vi "QAM_equalization.vi"() -> ()   [LabVIEW 2010]
doc: "This example demonstrates the implementation of Equalization in an QAM Modulation Demodulation System"
uses:
  <vilib>/AddOns/Modulation/Digital/General/MT Generate QAM System Parameters(M).vi
  <vilib>/measure/masml.llb/ma_sml_Interpolation by Zero Insert (complex input).vi
  <vilib>/addons/Modulation/Digital/General/MT Generate Bits (Galois, PN Order).vi
  <vilib>/AddOns/Modulation/Digital/General/MT Apply Matched Filter (Generic).vi
  <vilib>/AddOns/Modulation/Digital/General/MT Align to Ideal Symbols (Generic).vi
  <vilib>/AddOns/Modulation/Digital/Equalization/MT QAM Feedforward Equalizer (LMS) (Specify coefficients).vi
  <vilib>/AddOns/Modulation/Digital/Demodulation/MT Calculate BER After Trigger (PN Sequence).vi
  <vilib>/addons/Modulation/niDMT.lvlib
  <vilib>/Analysis/NI_AALBase.lvlib
  <vilib>/measure/NI_MAPro.lvlib
  <vilib>/AddOns/Modulation/Digital/General/MT Generate Symbol Map (Rectangular).vi
  <vilib>/AddOns/Modulation/Digital/General/MT Map Bits to QAM Symbols.vi
panel:
  out "pulse shaping filter coefficients":dbl[](graph)
  out "大小 5":i32
  out "大小 4":i32
  out "大小 3":i32
  out "大小 2":i32
  out "大小":i32
  out "Error Out":errorcluster
  in  "Error In":errorcluster
  in  "Reset?":bool
  out "Recovered":i8[](array[numeric])
  out "Message":i8[](array[numeric])
  in  "Equalizer length \n(symbols)":i32=48
  in  "PN Sequence Order":i32=26
  in  "Channel Filter Length\n(symbols)":i32=8
  out "BER Trigger Found Index (Bits)":u32
  out "Optimal Offset (Samples)":dbl format="%.4f"
  in  "Seed In":i32=-1
  out "Modulation Error Ratio (dB)":dbl format="%.2f"
  in  "Training Length\n(symbols)":i32=500
  in  "Channel Filter":T1(ring)=enum."Low-pass"
  out "BER":dbl format="%.4f"
  in  "Eb/N0 (10 dB)":dbl=50.0 format="%.2f"
  in  "Tab Control":T2(tab)=enum."RX Constellation (post equ)"
  in  "autoscale Tx":bool
  out "Constellation Graph (pre equ)":T3(graph)
  in  "Reset action":string="The example VI performs the following actions depending on the\nvalue of the boolean controls Reset? and Retrain Equalizer? :\n\n1. Reset?=TRUE: Reset all internal VIs,initialize equalizer coefficient array to equal the time-delayed dirac delta response {0 0 0... 1 ...0 0 0}, and feed training bits for equalization.\n\n2. Reset?=FALSE, Retrain Equalizer?=TRUE: Reset all receiver side VIs only,continue training the equalizer, and use final equalizer coefficient array from output of previous iteration as initial conditions for equalizer in current iteration\n\n3. Reset?=FALSE, Retrain Equalizer?=FALSE: Continue modulation, demodulation and equalization from previous iteration, while performing equalization in decision directed mode. This simulates the steady-state performance of the system once the equalizer error has fallen below a tolerance level."
  in  "autoscale Rx":bool
  out "Constellation Graph (post equ)":T3(graph)
  out "MER History":dbl(graph)=58.81121522824558
  out "LMS Error":dbl[](graph)
  out "Magnitude":dbl[][](graph)
  in  "Feedforward Equalizer (LMS)":T4={"Taps per Symbol"=1, "Delta (training)"=0.01, "Delta (steady state)"=0.01} {"Delta (steady state)" format="%#_6p"; "Delta (training)" format="%#_6p"}
  in  "Pulse Shaping Filter":T5(ring)=enum."Root Raised Cos"
  in  "Retrain\nEqualizer?":bool=TRUE
  in  "M-QAM Symbols":i32=1500
  in  "M-QAM":i32=256
  in  "Samples Per Symbol":i32=6
  in  "stop":bool
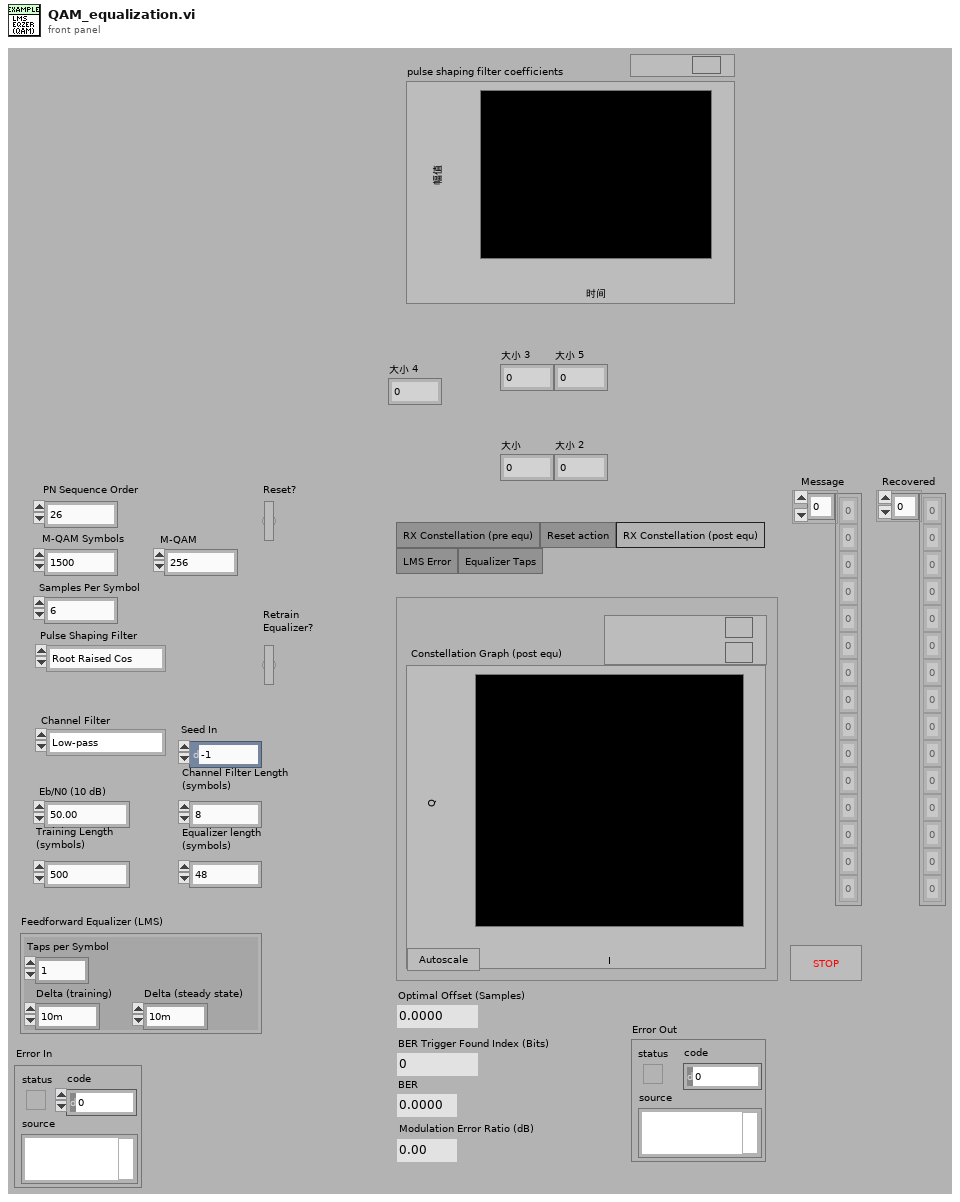
[diagram p1: front panel]
types:
  T1 = enum16{"Impulse", "Low-pass", "Custom filter", "Custom Filter-II"}
  T2 = enum32{"RX Constellation (pre equ)", "Reset action", "RX Constellation (post equ)", "LMS Error", "Equalizer Taps"}
  T3 = cluster{"Decimated Array":dbl[], "Decimated Array":dbl[]}[]
  T4 = cluster{"Taps per Symbol":i32, "Delta (training)":dbl, "Delta (steady state)":dbl}
  T5 = enum16{"none", "Raised Cosine", "Root Raised Cos", "Gaussian"}
  T6 = enum32{"None", "Hanning", "Hamming", "Triangular", "Blackman", "Exact Blackman", "Blackman-Harris", "Kaiser-Bessel", "Flat Top"}
  T7 = enum32{"Lowpass", "Highpass", "Bandpass", "Bandstop"}
  T8 = cluster{"start index (symbols)":i32, "width (symbols) (-1: all)":i32}
  T9 = cluster{"samples per symbol (16)":i32, "symbol map":cdb[]}
  T10 = typedef "niAMT.lvlib/Complex Data Waveform.ctl" = cluster{"t0":dbl, "dt":dbl, "Y":cdb[]}
  T11 = cluster{"constellation":dbl[], "oversampled data":dbl[]}[]
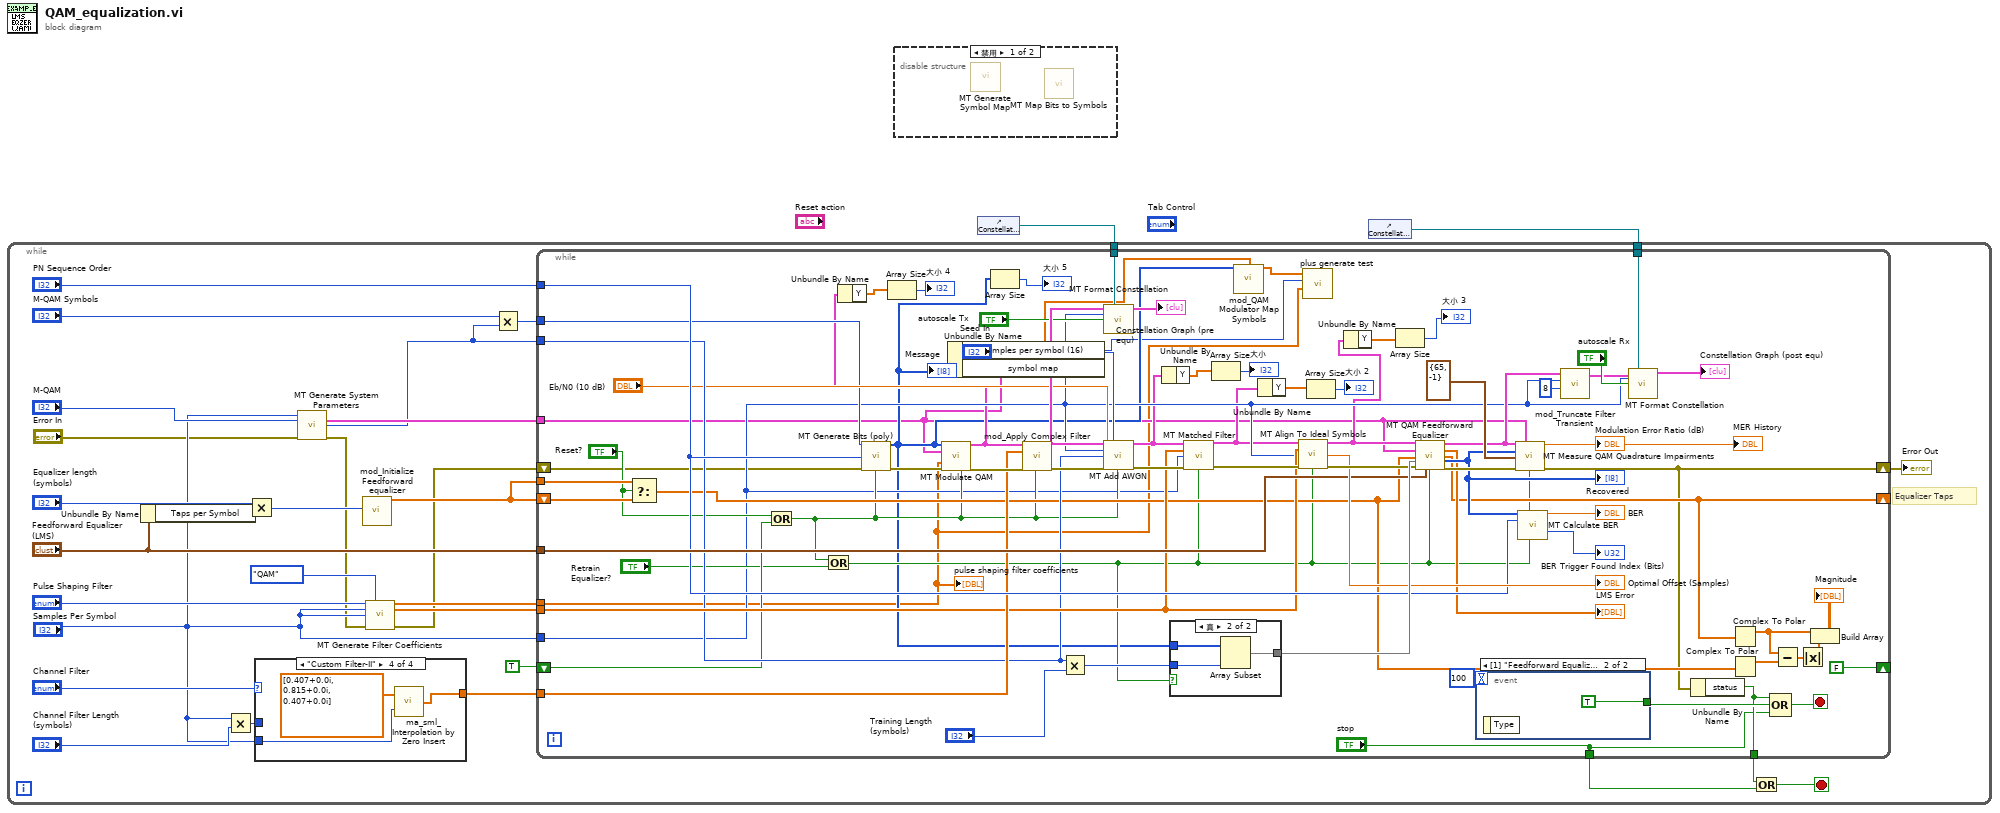
[diagram p0: block diagram]
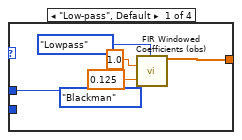
[diagram p3: hidden frame]
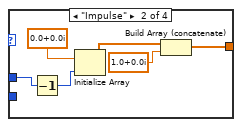
[diagram p4: hidden frame]
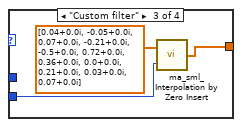
[diagram p5: hidden frame]
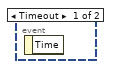
[diagram p7: hidden frame]
diagram:
  n1 = disable-structure shown="禁用" {
    frame Disabled {
      n2 = call-poly <vilib>:"MT Generate Symbol Map.vi"() -> ()  [unwired: 14 in, 2 out]
      n3 = call-poly <vilib>:"MT Map Bits to Symbols.vi"() -> ()  [unwired: 14 in, 2 out]
    }
    frame Enabled {
    }
  }
  n4 = control-ref of="Constellation Graph (pre equ)"() -> (w1:refnum<vi>)
  n5 = control-ref of="Constellation Graph (post equ)"() -> (w2:refnum<vi>)
  n6 = while {
    tunnel: w2 -> [w30]
    tunnel: w1 -> [w29]
    stop <- w5 stop-if-true
    # "Equalizer Taps"
    n7 = Unbundle By Name("Feedforward Equalizer (LMS)") -> ("Taps per Symbol"=w32:i32)
    n8 = Multiply(x="Samples Per Symbol", y="Channel Filter Length\n(symbols)") -> (x*y=w26:i32)
    n9 = Multiply(x="Equalizer length \n(symbols)", y=w32) -> (x*y=w10:i32)
    n10 = case shown="\"Custom Filter-II\"" "Channel Filter" {
      tunnel: [w34 w40 w46 w49] -> w22
      tunnel: w26 -> [w33 w39 _ _]
      tunnel: "Samples Per Symbol" -> [_ _ w45 w48]
      frame "Low-pass", Default {
        n11 = call <vilib>:"FIR Windowed Coefficients (obs).vi"("filter type"=T7."Lowpass", "sampling freq: fs"=1.0, "taps"=w33, "window"=T6."Blackman", "low cutoff freq: fl"=0.125) -> ("FIR Windowed Coefficients"=w34:dbl[])  [unwired: 2 in, 8 out]
      }
      frame "Impulse" {
        n12 = Decrement(x=w39) -> (x-1=w43:i32)
        n13 = Initialize Array(cdb 0.0+0.0i ("Element Data"), w43) -> (w42:cdb[])
        n14 = Build Array (concatenate)(w42, cdb 1.0+0.0i ("Element Data")) -> (w40:cdb[])
      }
      frame "Custom filter" {
        n15 = call-poly <vilib>:"ma_sml_Interpolation by Zero Insert.vi"("L"=w45, "x"=cdb[] [0.04+0.0i, -0.05+0.0i, 0.07+0.0i, -0.21+0.0i, -0.5+0.0i, 0.72+0.0i, 0.36+0.0i, 0.0+0.0i, 0.21+0.0i, 0.03+0.0i, 0.07+0.0i]) -> ("y"=w46:cdb[])
      }
      frame "Custom Filter-II" {
        n16 = call-poly <vilib>:"ma_sml_Interpolation by Zero Insert.vi"("L"=w48, "x"=cdb[] [0.407+0.0i, 0.815+0.0i, 0.407+0.0i]) -> ("y"=w49:cdb[])
      }
    }
    n17 = call-poly <vilib>:"MT Generate System Parameters.vi"("samples per symbol (16)"="Samples Per Symbol", "M-QAM (16)"="M-QAM", "error in (no error)"="Error In") -> ("QAM system parameters"=w21:T9, "bits per symbol"=w15:i32, "error out"=w9:errorcluster)  [unwired: 10 out]
    n18 = call <vilib>:"mod_Initialize Feedforward equalizer.vi"("tap length"=w10) -> ("equalizer taps"=w11:cdb[])  [unwired: 1 in, 13 out]
    n19 = call <vilib>:"MT Generate Filter Coefficients.vi"("pulse shaping filter (none)"="Pulse Shaping Filter", "modulation type"=enum16{"FSK", "PSK", "QAM", "MSK", "PAM", "ASK"}."QAM", "pulse shaping samples per symbol (16)"="Samples Per Symbol", "matched samples per symbol (16)"="Samples Per Symbol", "error in (no error)"=w9) -> ("pulse shaping filter coefficients"=w20:dbl[], "matched filter coefficients"=w19:dbl[], "error out"=w7:errorcluster)  [unwired: 2 in, 6 out]
    n20 = Multiply(x="M-QAM Symbols", y=w15) -> (x*y=w14:i32)
    n21 = while {
      shift-right: [w88] -> _
      shift-left: w11 -> [w93]
      tunnel: ["stop"] -> w6
      tunnel: "Feedforward Equalizer (LMS)" -> [w107]
      tunnel: w30 -> [w106]
      tunnel: w29 -> [w105]
      tunnel: "PN Sequence Order" -> [w104]
      tunnel: w15 -> [w101]
      tunnel: w22 -> [w103]
      tunnel: w21 -> [w55]
      tunnel: "Samples Per Symbol" -> [w76]
      tunnel: w20 -> [w52]
      tunnel: w19 -> [w102]
      tunnel: w14 -> [w97]
      tunnel: w11 -> [w92]
      shift-right: [FALSE] -> _
      shift-left: TRUE -> [w80]
      shift-right: [w74] -> w3
      shift-left: w7 -> [w75]
      tunnel: [w71] -> w4
      stop <- w72 stop-if-true
      n22 = Select(t=w92, s="Reset?", f=w93) -> (s? t:f=w87:cdb[])
      n23 = Or(x="Reset?", y=w80) -> (x .or. y?=w79:bool)
      n24 = Or(x=w79, y="Retrain\nEqualizer?") -> (x .or. y?=w78:bool)
      n25 = call-poly <vilib>:"MT Generate Bits (poly).vi"("total bits (128)"=w97, "PN sequence order (9)"=w104, "error in (no error)"=w75, "reset? (T)"=w79) -> ("output bit stream"=w56:i8[], "error out"=w126:errorcluster)  [unwired: 1 in, 9 out]
      "Message" <- w56
      n26 = call <vilib>:"MT Modulate QAM.vi"("input bit stream"=w56, "QAM system parameters"=w55, "pulse shaping filter coefficients"=w52, "error in (no error)"=w126, "reset? (T)"=w79) -> ("output complex waveform"=w58:T10, "error out"=w125:errorcluster)  [unwired: 2 in, 7 out]
      n27 = Unbundle By Name(w58) -> ("Y"=w59:cdb[])
      n28 = Array Size(array=w59) -> (size(s)=→"大小 4":i32)
      n29 = Unbundle By Name(w55) -> ("samples per symbol (16)"=w51:i32, "symbol map"=w54:cdb[])
      n30 = Array Size(array=w56) -> (size(s)=→"大小 5":i32)
      n31 = call <vilib>:"mod_Apply Complex Filter.vi"("input complex waveform"=w58, "filter coefficients"=w103, "reset? (T)"=w79, "error in (no error)"=w125) -> ("output complex waveform"=w123:cluster{"t0":dbl, "dt":dbl, "Y":cdb[]}, "error out"=w119:errorcluster)  [unwired: 10 out]
      n32 = Multiply(x=w101, y="Training Length\n(symbols)") -> (x*y=w115:i32)
      n33 = call <vilib>:"MT Format Constellation.vi"("waveform"=w123, "constellation reference"=w105, "samples per symbol"=w76, "autoscale"="autoscale Tx") -> ("constellation graph"=→"Constellation Graph (pre equ)":T11)  [unwired: 1 in, 10 out]
      n34 = call <vilib>:"MT Add AWGN.vi"("input complex waveform"=w123, "samples per symbol (16)"=w76, "bits per symbol (1)"=w101, "Eb/N0 (10 dB)"="Eb/N0 (10 dB)", "error in (no error)"=w119, "seed in (0xFFFFFFFF)"="Seed In", "reset? (T)"=w79) -> ("output complex waveform"=w69:T10, "error out"=w118:errorcluster)  [unwired: 7 out]
      n35 = Unbundle By Name(w69) -> ("Y"=w67:cdb[])
      n36 = case shown="真" w78 {
        tunnel: w56 -> [_ w130]
        tunnel: w115 -> [_ w129]
        tunnel: [_ w128] -> w116
        frame False {
        }
        frame True {
          n37 = Array Subset(array=w130, length=w129) -> (w128:i8[])  [unwired: 1 in]
        }
      }
      n38 = call-poly <vilib>:"MT Matched Filter.vi"("input complex waveform"=w69, "matched filter coefficients"=w102, "samples per symbol (16)"=w76, "error in (no error)"=w118, "reset? (T)"=w78) -> ("output complex waveform"=w68:T10, "error out"=w110:errorcluster)  [unwired: 9 out]
      n39 = Array Size(array=w67) -> (size(s)=→"大小":i32)
      n40 = call <vilib>:"mod_QAM Modulator Map Symbols.vi"("Input Bit Stream"=w56, "Symbol Map"=w54) -> ("Symbols"=w53:cdb[])  [unwired: 2 in, 11 out]
      n41 = Unbundle By Name(w68) -> ("Y"=w65:cdb[])
      n42 = call-poly <vilib>:"MT Align To Ideal Symbols.vi"("input complex waveform"=w68, "matched filter coefficients"=w102, "samples per symbol (16)"=w76, "error in (no error)"=w110, "reset? (T)"=w78) -> ("output complex waveform"=w63:T10, "waveform alignment offset (samples)"=→"Optimal Offset (Samples)":dbl, "error out"=w109:errorcluster)  [unwired: 8 out]
      n43 = call "plus generate test.vi"("Pulse Shaping Filter Coefficients"=w52, "Samples Per Symbol (16)"=w51, "Symbols"=w53) -> ()  [unwired: 8 in, 1 out]
      n44 = Array Size(array=w65) -> (size(s)=→"大小 2":i32)
      n45 = Unbundle By Name(w63) -> ("Y"=w62:cdb[])
      n46 = Array Size(array=w62) -> (size(s)=→"大小 3":i32)
      n47 = call-poly <vilib>:"MT QAM Feedforward Equalizer.vi"("input complex waveform"=w63, "QAM system parameters"=w55, "equalizer coefficients in"=w87, "training bits"=w116, "error in (no error)"=w109, "feedforward equalizer (LMS) parameters"=w107, "reset? (T)"=w78) -> ("output complex waveform"=w96:T10, "error (V^2)"=→"LMS Error":dbl[], "equalizer coefficients out"=w88:cdb[], "output bit stream"=w99:i8[], "error out"=w111:errorcluster)  [unwired: 4 out]
      "Recovered" <- w99
      n48 = event shown="[1] \"Feedforward Equalizer (LMS)\", \"Equalizer length \n(symbols)\", \"Channel Filter\", \"Channel Filter Length\n(symbols)\", \"M-QAM\", \"Samples Per Symbol\", \"Pulse Shaping Filter\": 值改变" {
        selector: _ -> [_ _]
        dyn-events: _ -> [_ _]
        timeout: 100 -> [_ _]
        tunnel: [_ TRUE ("stop")] -> w73
        event Timeout {
          n49 = event-data() -> ()  [unwired: 2 out]
        }
        event "Feedforward Equalizer (LMS)", "Equalizer length \n(symbols)", "Channel Filter", "Channel Filter Length\n(symbols)", "M-QAM", "Samples Per Symbol", "Pulse Shaping Filter": Value Change {
          n50 = event-data() -> ()  [unwired: 2 out]
        }
      }
      n51 = call <vilib>:"MT Measure QAM Quadrature Impairments.vi"("recovered complex waveform"=w96, "QAM system parameters"=w55, "input bit stream"=w99, "impairment measurement window"=T8 {"start index (symbols)"=65, "width (symbols) (-1: all)"=-1}, "error in (no error)"=w111, "reset? (T)"=w78) -> ("modulation error ratio (dB)"=→"Modulation Error Ratio (dB)" →"MER History":dbl, "error out"=w74:errorcluster)  [unwired: 1 in, 7 out]
      n52 = call-poly <vilib>:"MT Calculate BER.vi"("input bit stream"=w99, "PN sequence order (9)"=w104, "reset? (T)"=w78) -> ("BER"=→"BER":dbl, "trigger found index (bits)"=→"BER Trigger Found Index (Bits)":u32)  [unwired: 3 in, 8 out]
      n53 = call <vilib>:"mod_Truncate Filter Transient.vi"("filter length (sym)"=8, "samples/symbol"=w76, "input complex waveform"=w96) -> ("output complex waveform"=w95:T10)  [unwired: 8 out]
      n54 = call <vilib>:"MT Format Constellation.vi"("waveform"=w95, "constellation reference"=w106, "samples per symbol"=w76, "autoscale"="autoscale Rx") -> ("constellation graph"=→"Constellation Graph (post equ)":T11)  [unwired: 1 in, 10 out]
      n55 = Unbundle By Name(w74) -> ("status"=w71:bool)
      n56 = Complex To Polar(r * e^(i*theta)=w88) -> (r=w85:dbl[])  [unwired: 1 out]
      n57 = Complex To Polar(r * e^(i*theta)=w87) -> (r=w84:dbl[])  [unwired: 1 out]
      n58 = Compound Arithmetic op=OR(w71, w73, "stop") -> (w72:bool)
      n59 = Subtract(x=w85, y=w84) -> (x-y=w83:dbl[])
      n60 = Absolute Value(x=w83) -> (abs(x)=w82:dbl[])
      n61 = Build Array(w85, w82) -> (→"Magnitude":dbl[][])
      "pulse shaping filter coefficients" <- w52
    }
    "Error Out" <- w3
    n62 = Or(x=w4, y=w6) -> (x .or. y?=w5:bool)
  }
